vi "Update_List_Symbol.vi"(10 "current sample":u16, 11 "MulticolumnListbox in":refnum<vi>) -> ()   [LabVIEW 2013]
doc: "Updates the symbol of the currently running sample to a checkmark"
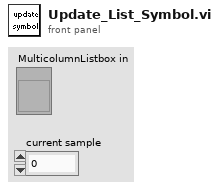
[diagram p1: front panel]
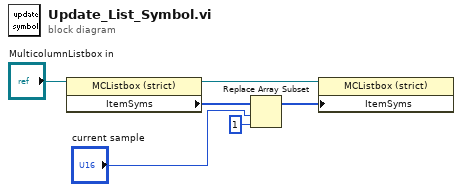
[diagram p0: block diagram]
diagram:
  n1 = property on="Property Node" class="MCListbox (strict)"(reference="MulticolumnListbox in") -> (reference out=w2:refnum<vi>, "ItemSyms"=w4:i32[])  [unwired: 1 in, 1 out]
  n2 = Replace Array Subset(array=w4, new element=1 ("new element/subarray"), index="current sample") -> (w6:i32[])
  n3 = property on="Property Node" class="MCListbox (strict)"(reference=w2, "ItemSyms"=w6) -> ()  [unwired: 1 in, 2 out]
